vi "Find OOB Server Ports.vi"(8 "error in":errorcluster) -> (3 "Ports":u16[](array[numeric]))   [LabVIEW 2026]
uses:
  <vilib>/Utility/error.llb/Trim Whitespace One-Sided.vi
panel:
  out "netstat":T1(array[cluster])
  out "standard error":string
  out "return code":i32
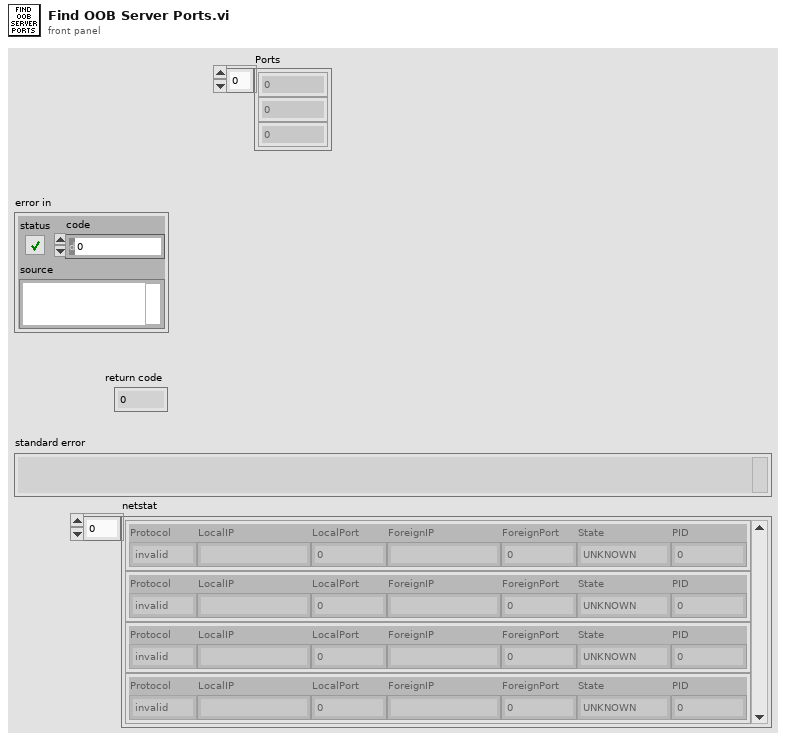
[diagram p1: front panel]
types:
  T1 = cluster{"Protocol":enum16{"invalid", "tcp", "udp", "icmp", "ip", "tcpv6", "udpv6", "icmpv6", "ipv6"}, "LocalIP":string, "LocalPort":u16, "ForeignIP":string, "ForeignPort":u16, "State":enum8{"UNKNOWN", "LISTEN", "ESTABLISHED", "SYN_SENT", "SYN_RECV", "LAST_ACK", "CLOSE_WAIT", "TIME_WAIT", "CLOSED", "CLOSING", "FIN_WAIT1", "FIN_WAIT2"}, "PID":u16}[]
  T2 = enum8{"UNKNOWN", "LISTEN", "ESTABLISHED", "SYN_SENT", "SYN_RECV", "LAST_ACK", "CLOSE_WAIT", "TIME_WAIT", "CLOSED", "CLOSING", "FIN_WAIT1", "FIN_WAIT2"}
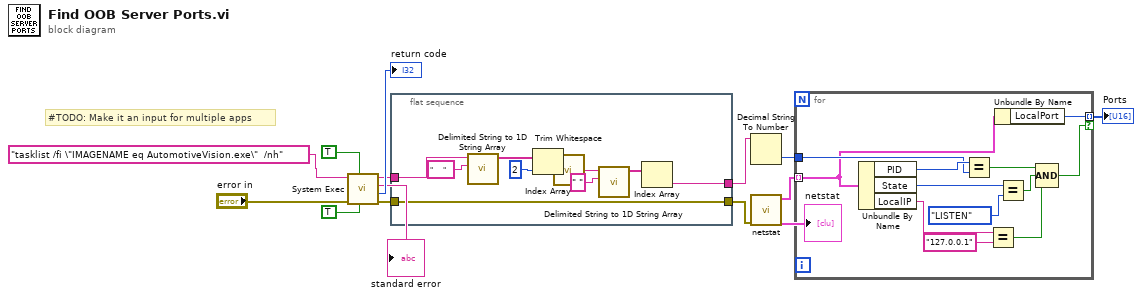
[diagram p0: block diagram]
diagram:
  # "#TODO: Make it an input for multiple apps"
  n1 = call <vilib>:"System Exec.vi"("run minimized? (F)"=TRUE, "wait until completion? (T)"=TRUE, "error in (no error)"="error in", "command line"="tasklist /fi \"IMAGENAME eq AutomotiveVision.exe\"  /nh") -> ("error out"=w9:errorcluster, "return code"=→"return code":i32, "standard error"=→"standard error":string, "standard output"=w7:string)  [unwired: 4 in]
  n2 = flat-sequence {
    tunnel: w7 -> [w23]
    tunnel: [w16] -> w8
    tunnel: w9 -> [w15]
    tunnel: [w15] -> w4
    frame #0 {
      n3 = call <vilib>:"Delimited String to 1D String Array.vi"("delimiter"="     ", "delimited string"=w23) -> ("string array"=w21:string[])  [unwired: 9 in]
      n4 = Index Array(array=w21, index=2) -> (element=w19:string)
      n5 = call <vilib>:"Trim Whitespace.vi"("string"=w19) -> ("trimmed string"=w14:string)  [unwired: 1 in]
      n6 = call <vilib>:"Delimited String to 1D String Array.vi"("delimiter"=" ", "delimited string"=w14) -> ("string array"=w17:string[])  [unwired: 9 in]
      n7 = Index Array(array=w17) -> (element=w16:string)  [unwired: 1 in]
    }
  }
  n8 = Decimal String To Number(string=w8) -> (number=w6:i32)  [unwired: 2 in, 1 out]
  n9 = call "netstat.vi"("error in (no error)"=w4) -> ("netstat"=w5:T1)  [unwired: 9 in, 1 out]
  "netstat" <- w5
  n10 = for {
    tunnel: w5 -> [w26] mode=indexing
    tunnel: w6 -> [w34]
    tunnel: [w25] -> w3 mode=indexing if=w24
    n11 = Unbundle By Name(w26) -> ("PID"=w35:u16, "State"=w32:T2, "LocalIP"=w29:string)
    n12 = Equal?(x=w35, y=w34) -> (x = y?=w33:bool)
    n13 = Equal?(x=w29, y="127.0.0.1") -> (x = y?=w27:bool)
    n14 = Unbundle By Name(w26) -> ("LocalPort"=w25:u16)
    n15 = Equal?(x=w32, y=T2."LISTEN") -> (x = y?=w30:bool)
    n16 = Compound Arithmetic op=AND(w33, w30, w27) -> (w24:bool)
  }
  "Ports" <- w3
